vi "ShowDetailResult.vi"(8 "error in (no error)":errorcluster caption="错误输入（无错误）", 11 "DataBase in":refnum<class "DataBase.lvclass">) -> (0 "error out":errorcluster caption="错误输出", 3 "DataBase out":refnum<class "DataBase.lvclass">)   [LabVIEW 2019, in "DataBase.lvlib" / "DataBase.lvclass"]
uses:
  DataBase.lvclass
  DataBase.lvclass/DataBase.ctl
  <vilib>/Utility/miscctls.llb/LVRowAndColumnTypeDef.ctl
  <vilib>/Utility/file.llb/Read Delimited Spreadsheet (string).vi
panel:
  out "File Path Indicator":path
  in  "Multicolumn Listbox":i32(listbox)
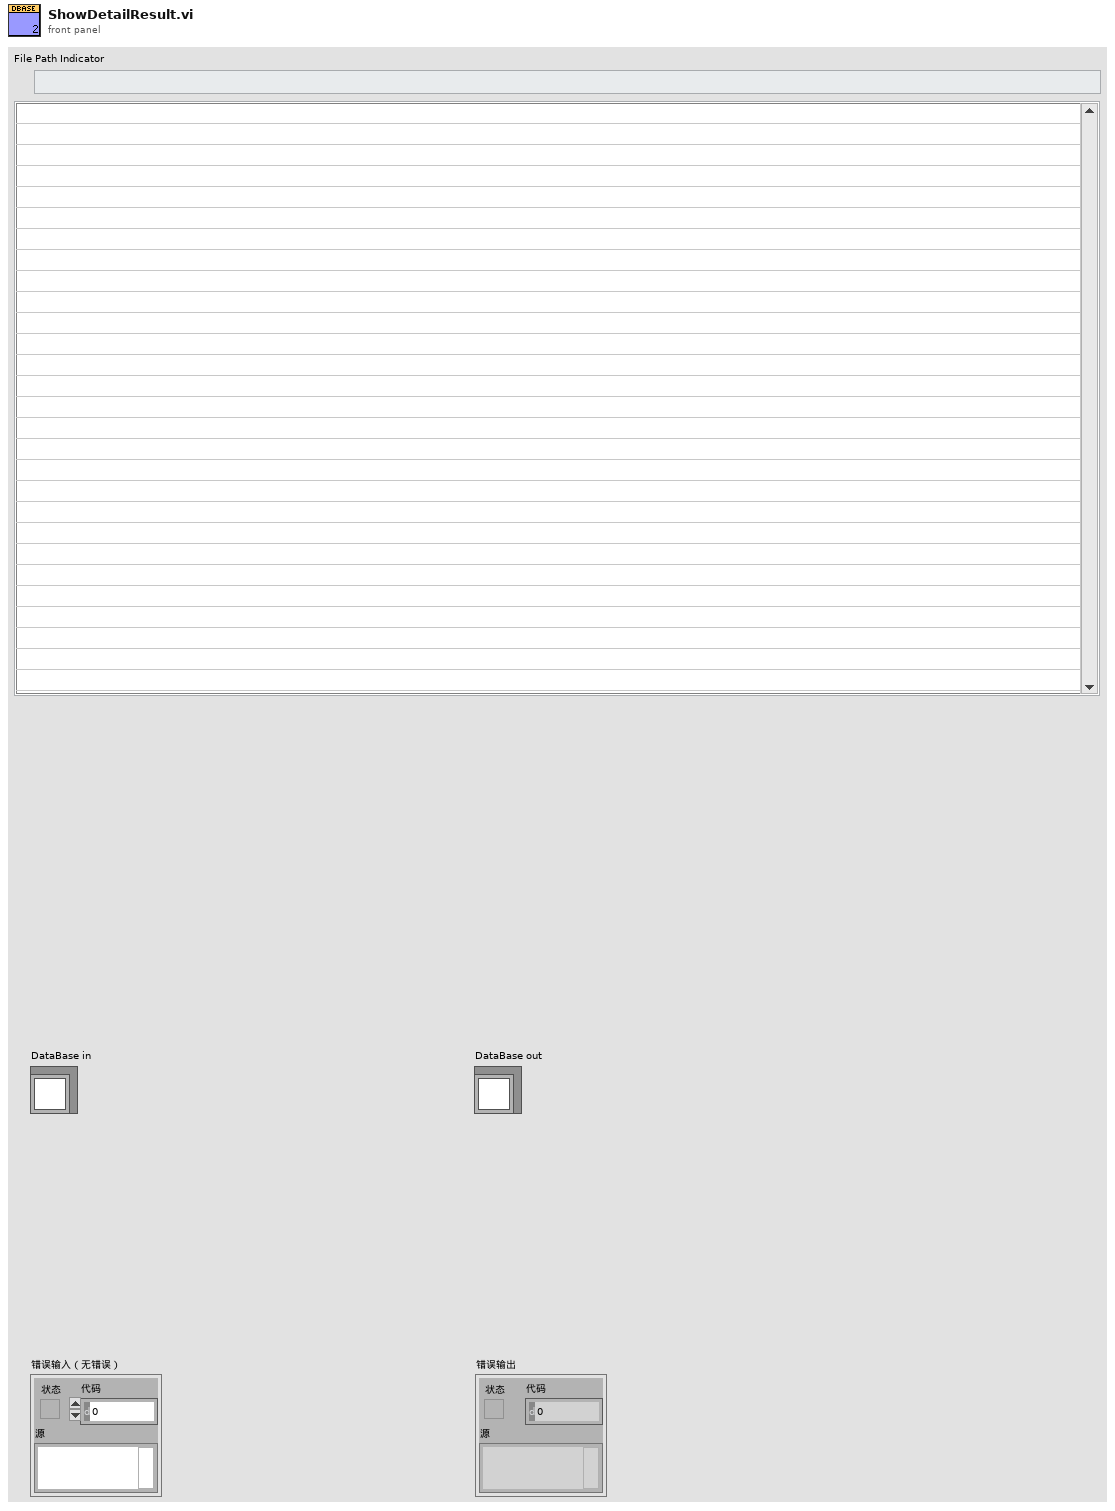
[diagram p1: front panel]
types:
  T1 = enum32{"Invalid", "Standard", "Closed", "Hidden", "Minimized", "Maximized"}
  T2 = enum32{"invalid app kind", "Development System", "Run Time System", "Student Edition", "Embedded LabVIEW", "Evaluation", "Custom"}
  T3 = typedef "LVRowAndColumnTypeDef.ctl" = cluster{"Row":i32, "Column":i32}
  T4 = cluster{"Core":cluster{"Current VI Reference":refnum<vi>, "Close Panel on Exit?":bool}, "Your Boolean data":bool, "Your string data":string, "Multicolumn Listbox":refnum<vi>}
  T5 = cluster{"Current VI Reference":refnum<vi>, "Close Panel on Exit?":bool}
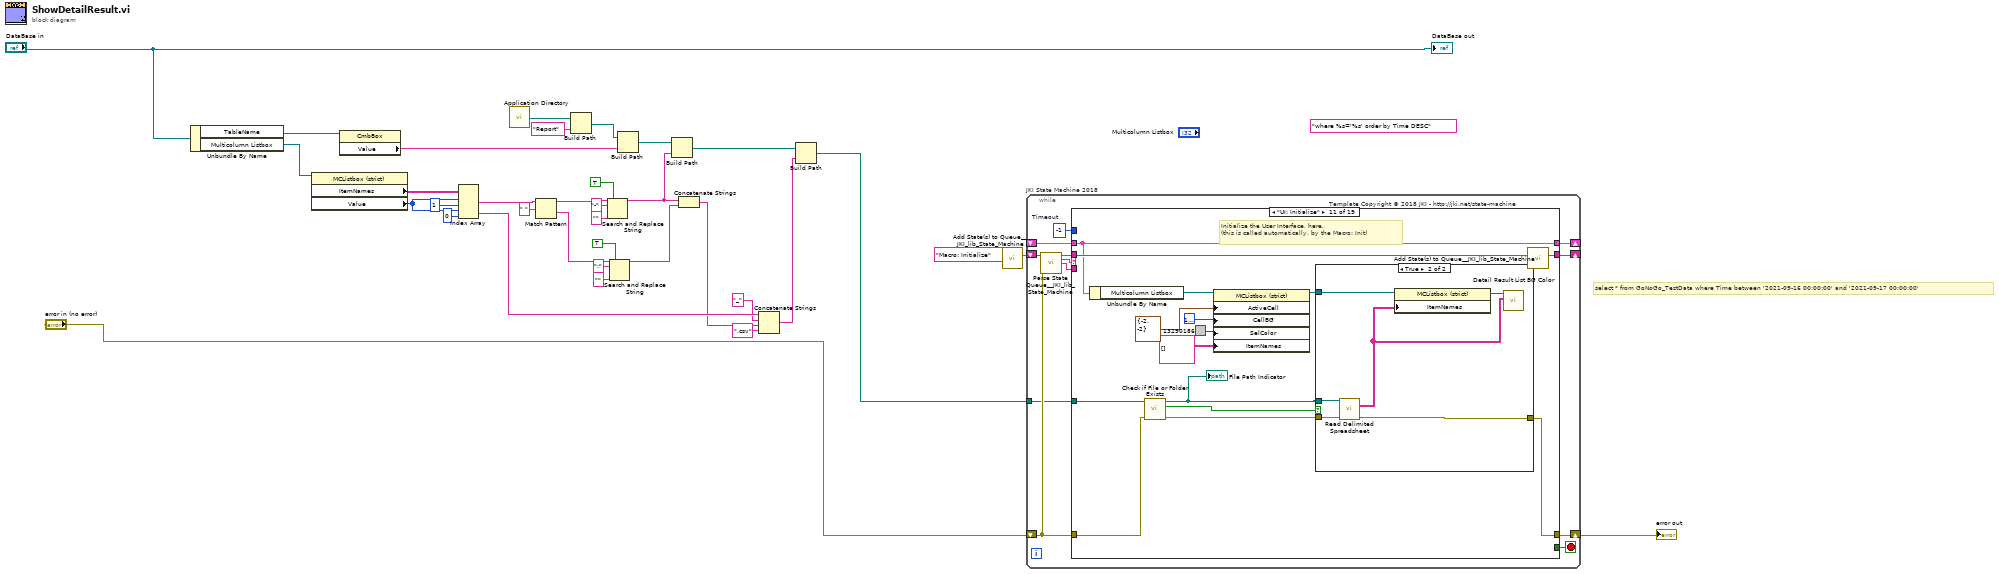
[diagram p0: block diagram]
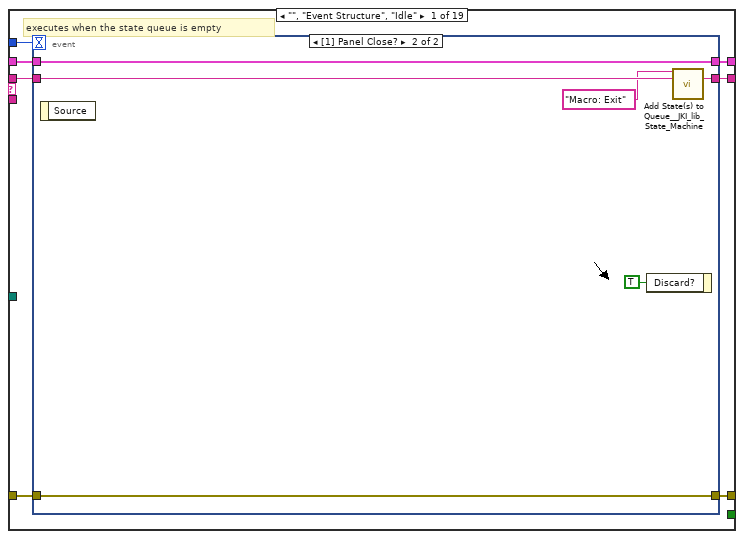
[diagram p2: hidden frame]
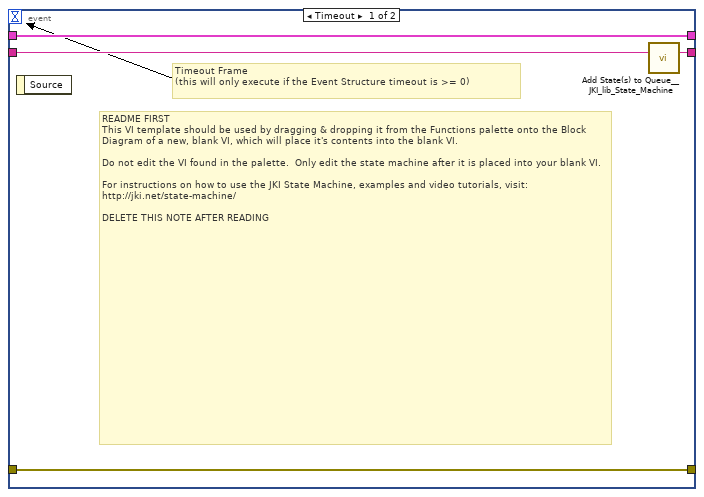
[diagram p3: hidden frame]
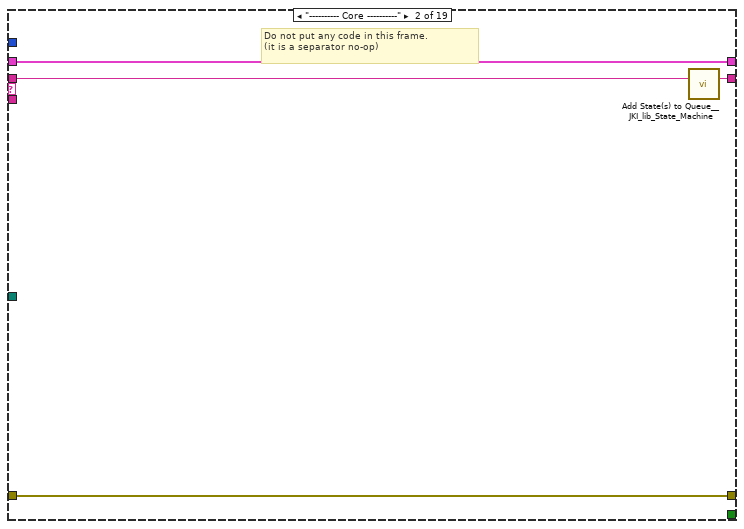
[diagram p4: hidden frame]
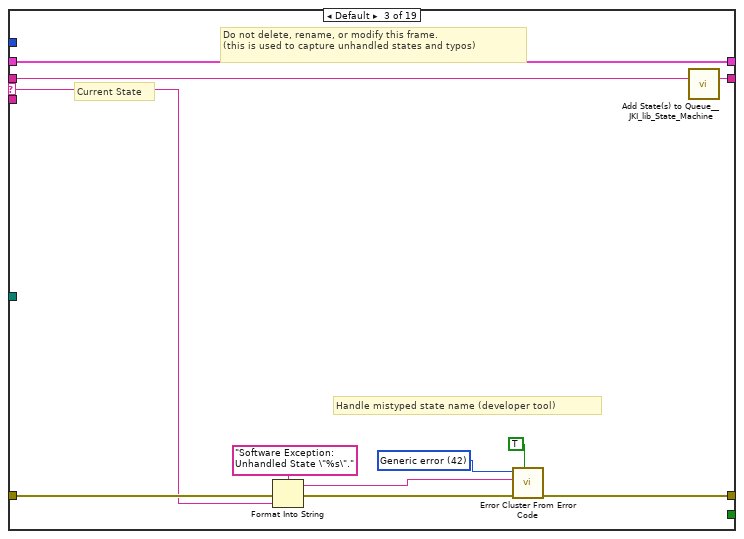
[diagram p5: hidden frame]
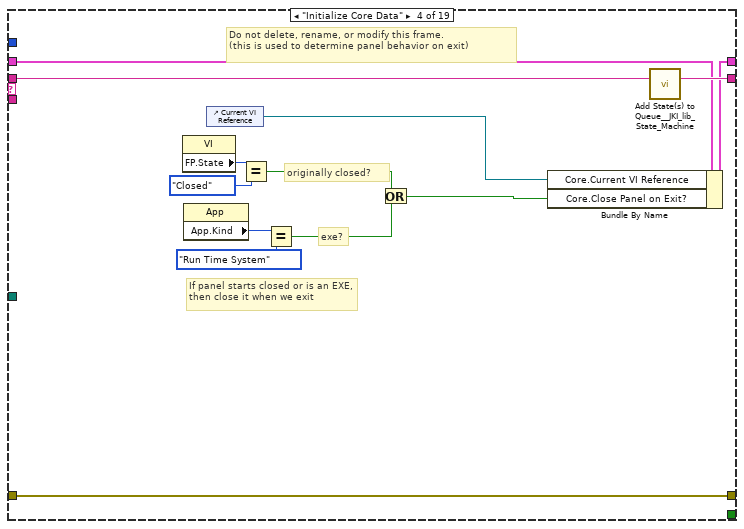
[diagram p6: hidden frame]
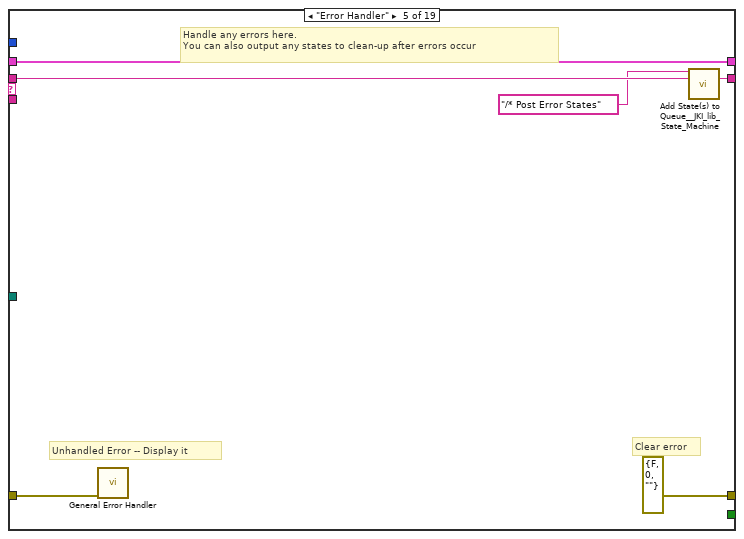
[diagram p7: hidden frame]
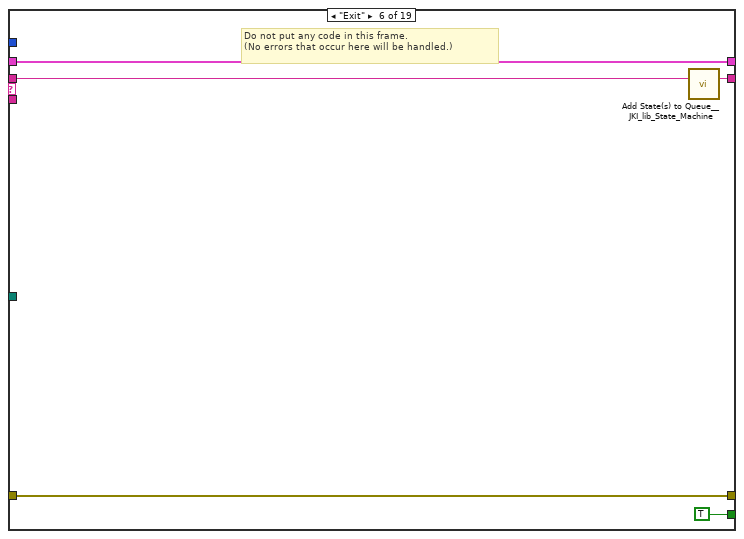
[diagram p8: hidden frame]
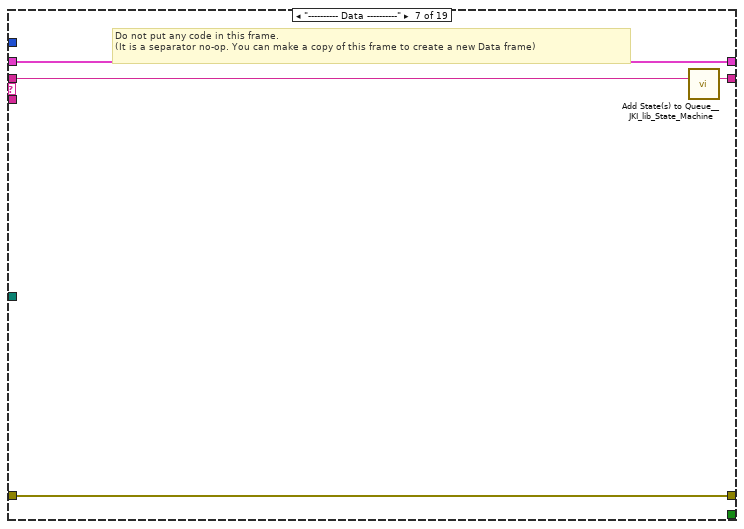
[diagram p9: hidden frame]
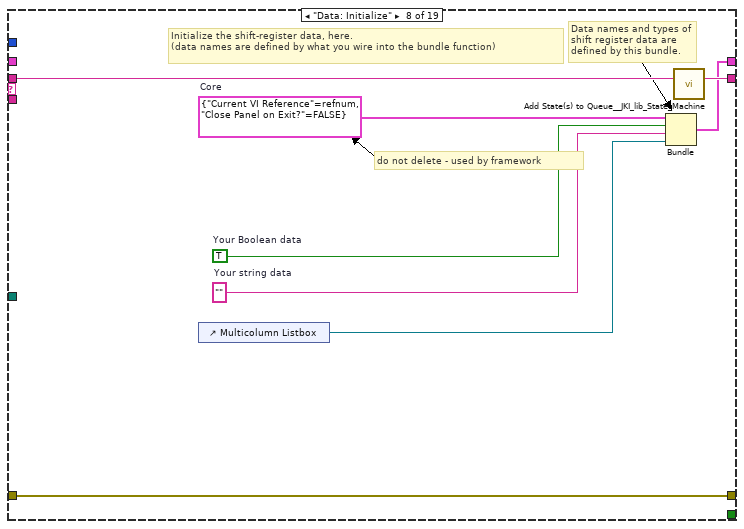
[diagram p10: hidden frame]
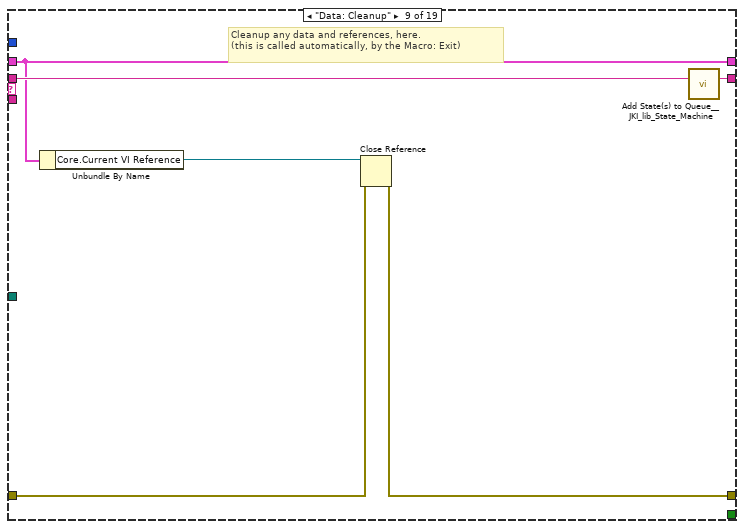
[diagram p11: hidden frame]
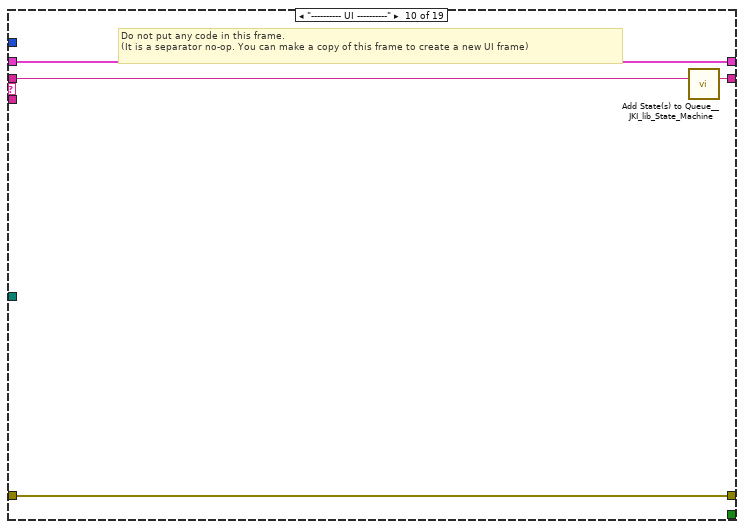
[diagram p12: hidden frame]
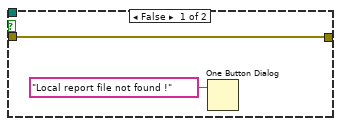
[diagram p13: hidden frame]
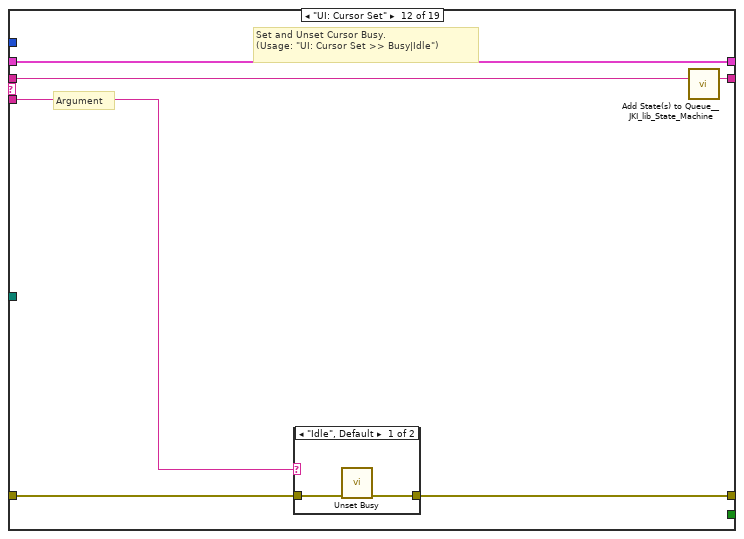
[diagram p14: hidden frame]
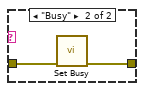
[diagram p15: hidden frame]
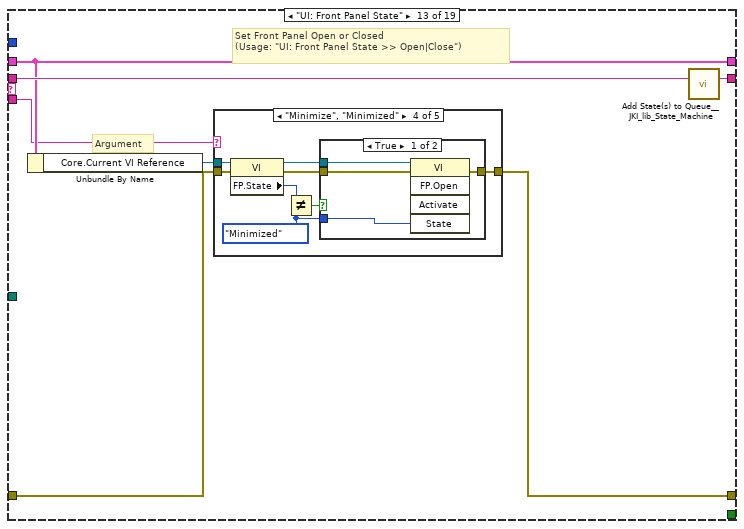
[diagram p16: hidden frame]
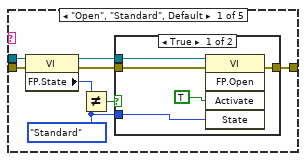
[diagram p17: hidden frame]
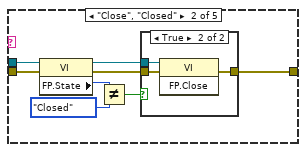
[diagram p19: hidden frame]
diagram:
  (unwired) "where %s='%s' order by Time DESC" ("format string")
  # "select * from GoNoGo_TestData where Time between '2021-09-16 00:00:00' and '2021-09-17 00:00:00'"
  n1 = Unbundle By Name("DataBase in") -> ("TableName"=w32:refnum<vi>, "Multicolumn Listbox"=w26:refnum<vi>)
  n2 = property class="MCListbox (strict)"(reference=w26) -> ("ItemNames"=w25:string[][], "Value"=w16:i32)  [unwired: 1 in, 2 out]
  n3 = property class="CmbBox"(reference=w32) -> ("Value"=w28:string)  [unwired: 1 in, 2 out]
  n4 = Index Array(array=w25, index (row) #1=w16, index (col) #1=1 ("disabled index (col)"), index (row) #2=w16, index (col) #2=0 ("disabled index (col)")) -> (element #1=w22:string, element #2=w8:string)
  n5 = call <vilib>:"Application Directory.vi"() -> ("Application Directory"=w31:path)
  n6 = Match Pattern(string=w22, regular expression=" ") -> (before substring=w21:string, after substring=w11:string)  [unwired: 1 in, 2 out]
  n7 = Build Path(base path=w31, name or relative path="Report") -> (appended path=w30:path)
  n8 = Search and Replace String(replace all?=TRUE ("replace all? (F)"), input string=w21, search string="-", replace string="" ("replace string (\"\")")) -> (result string=w10:string)  [unwired: 4 in, 3 out]
  n9 = Search and Replace String(replace all?=TRUE ("replace all? (F)"), input string=w11, search string=":", replace string="" ("replace string (\"\")")) -> (result string=w9:string)  [unwired: 4 in, 3 out]
  n10 = Build Path(base path=w30, name or relative path=w28) -> (appended path=w27:path)
  n11 = Build Path(base path=w27, name or relative path=w10) -> (appended path=w17:path)
  n12 = Concatenate Strings(w10, w9) -> (w6:string)
  n13 = Concatenate Strings(w8, "_" ("string"), w6, ".csv" ("string")) -> (w4:string)
  n14 = Build Path(base path=w17, name or relative path=w4) -> (appended path=w1:path)
  n15 = call <vilib>:"Add State(s) to Queue__JKI_lib_State_Machine.vi"("State(s) in (\"\")"="Macro: Initialize") -> ("States Out"=w34:string)  [unwired: 14 in]
  n16 = while "JKI State Machine 2018" {
    shift-right: [w40] -> _
    shift-left: _ -> [w39]
    shift-right: [w43] -> w2
    shift-left: "error in (no error)" -> [w37]
    shift-right: [w42] -> _
    shift-left: w34 -> [w44]
    tunnel: w1 -> [w36]
    stop <- w41 stop-if-true
    w38 = -1  # Timeout
    # "Template Copyright © 2018 JKI - http://jki.net/state-machine"
    n17 = call <vilib>:"Parse State Queue__JKI_lib_State_Machine.vi"("State Queue"=w44, "Error In (no error)"=w37) -> ("Remaining States"=w46:string, "Current State"=w47:string, "Arguments"=w45:string)  [unwired: 11 in]
    n18 = case shown="\"UI: Initialize\"" w47 {
      selector: w47 -> [_ _ w69 _ _ _ _ _ _ _ _ _ _ _ _ _ _ _ _]
      tunnel: w46 -> [w54 w68 w73 w92 w98 w103 w107 w115 w121 w125 w140 w154 w165 w234 w239 w249 w253 w257 w261]
      tunnel: w45 -> [_ _ _ _ _ _ _ _ _ _ _ w149 w159 _ _ _ _ _ _]
      tunnel: w39 -> [w52 w65 w71 w85 w95 w101 w104 _ w116 w122 w135 w152 w161 w231 w236 w246 w250 w254 w258]
      tunnel: [w51 w66 w75 w89 errorcluster {"status"=FALSE, "code"=0, "source"=""} ("error out") w100 w105 w112 w117 w123 w132 w150 w162 w232 w237 w247 w251 w255 w259] -> w43
      tunnel: w37 -> [w50 w66 w74 w89 w94 w100 w105 w112 w118 w123 w133 w151 w163 w232 w237 w247 w251 w255 w259]
      tunnel: [w53 w67 w72 w91 w97 w102 w106 w114 w120 w124 w139 w153 w164 w233 w238 w248 w252 w256 w260] -> w42
      tunnel: [_ _ _ _ _ TRUE _ _ _ _ _ _ _ _ _ _ _ _ _] -> w41
      tunnel: [w49 w65 w71 w90 w95 w101 w104 w113 w116 w122 w135 w152 w161 w231 w236 w246 w250 w254 w258] -> w40
      tunnel: w38 -> [w48 _ _ _ _ _ _ _ _ _ _ _ _ _ _ _ _ _ _]
      tunnel: w36 -> [_ _ _ _ _ _ _ _ _ _ w134 _ _ _ _ _ _ _ _]
      frame "", "Event Structure", "Idle" {
        # "executes when the state queue is empty"
        n19 = event shown="[1] Panel Close?" {
          selector: _ -> [_ _]
          dyn-events: _ -> [_ _]
          timeout: w48 -> [_ _]
          tunnel: w54 -> [w58 w64]
          tunnel: [w57 w63] -> w53
          tunnel: w52 -> [w55 w61]
          tunnel: [w56 w62] -> w51
          tunnel: w50 -> [w56 w62]
          tunnel: [w55 w61] -> w49
          event Timeout {
            # "README FIRST\nThis VI template should be used by dragging & dropping it from the Functions palette onto the Block Diagram of a new, blank VI, which will place it's contents into the blank VI.\n\nDo not edit the VI found in the palette.  Only edit the state machine after it is placed into your blank VI.\n\nFor instructions on how to use the JKI State Machine, examples and video tutorials, visit:\nhttp://jki.net/state-machine/\n\nDELETE THIS NOTE AFTER READING"
            # "Timeout Frame\n(this will only execute if the Event Structure timeout is >= 0)"
            n20 = event-data() -> ()  [unwired: 1 in, 1 out]
            n21 = call <vilib>:"Add State(s) to Queue__JKI_lib_State_Machine.vi"("State(s) in (\"\")"=w58) -> ("States Out"=w57:string)  [unwired: 14 in]
          }
          event Panel Close? {
            n22 = event-data() -> ()  [unwired: 1 in, 1 out]
            n23 = event-data("Discard?"=TRUE) -> ()  [unwired: 1 in, 1 out]
            n24 = call <vilib>:"Add State(s) to Queue__JKI_lib_State_Machine.vi"("State(s) in Front (\"\")"="Macro: Exit", "State(s) in (\"\")"=w64) -> ("States Out"=w63:string)  [unwired: 13 in]
          }
        }
      }
      frame "---------- Core ----------" {
        # "Do not put any code in this frame.\n(it is a separator no-op)"
        n25 = call <vilib>:"Add State(s) to Queue__JKI_lib_State_Machine.vi"("State(s) in (\"\")"=w68) -> ("States Out"=w67:string)  [unwired: 14 in]
      }
      frame Default {
        w78 = 42 items=["No error", "Argument error", "Memory is full", "Out of zone", "End of file", "File already open", "Generic file I/O error", "File not found", "File permission error", "Disk is full", "Duplicate path", "Too many files open", "System feature not enabled", "Resource file not found", "Cannot add resource", "Resource not found", "Image not found", "Image memory error", "Pen does not exist", "Config type invalid", "Config token not found", "Config parse error", "Config memory error", "Bad external code format", "Bad external code offset", "External code not present", "Null window", "Destroy window error", "Null menu", "Print aborted", "Bad print record", "Print driver error", "Windows error during printing", "Memory error during printing", "Print dialog error", "Generic print error", "Invalid device refnum", "Device not found", "Device parameter error", "Device unit error", "Cannot open device", "Device call aborted", "Generic error", "Cancelled by user", "Object ID too low", "Object ID too high", "Object not in heap", "Unknown heap", "Unknown object (invalid DefProc)", "Unknown object (DefProc not in table)", "Message out of range", "Invalid (null) method", "Unknown message", "Manager call not supported", "Bad address", "Network operation in progress", "Network operation timed out", "Connection is busy", "Network attribute not supported", "Network error", "Address in use", "System out of memory", "Connection aborted", "Connection refused", "Not connected", "Already connected", "Connection closed", "Initialization error (interapplication manager)", "Bad occurrence", "Wait on unbound occurrence handler", "Occurrence queue overflow", "Datalog type conflict", "Unused", "Unrecognized type (interapplication manager)", "Memory corrupt", "Failed to make temporary DLL", "Old CIN version", "Drag socket not found", "Failed to load drop-object", "Failed to register OLE object", "Failed to release OLE object", "Format specifier type mismatch", "Unknown format specifier", "Too few format specifiers", "Too many format specifiers", "Scan failed", "Newer CIN version", "Error converting to variant", "Runtime menu error", "Password tampered", "Variant attribute not found", "Incompatible variant data type", "Event data is not available", "Event Store is not present", "Occurrence is not found", "Event Queue is not created", "Event info is not available", "Refnum passed is NULL", "Error retrieving Class GUID", "Error retrieving CoClass GUID", "Error retrieving TypeLib GUID.", "Bad built application magic bytes.", "Specific driver is different from the specific driver associated with the Logical Name.", "There is no session opened to the class driver.", "Max Error", "MAX - Error with config objects", "MAX - Error loading configuration", "MAX - Group not supported"]
        # "Current State"
        # "Do not delete, rename, or modify this frame.\n(this is used to capture unhandled states and typos)"
        # "Handle mistyped state name (developer tool)"
        n26 = Format Into String(format string="Software Exception: Unhandled State \"%s\"." ("message"), error in=w74, w69) -> (resulting string=w77:string, error out=w76:errorcluster)  [unwired: 1 in]
        n27 = call <vilib>:"Error Cluster From Error Code.vi"("show call chain? (False)"=TRUE, "error in (no error)"=w76, "error message (\"\")"=w77, "error code (0)"=w78) -> ("error out"=w75:errorcluster)  [unwired: 5 in]
        n28 = call <vilib>:"Add State(s) to Queue__JKI_lib_State_Machine.vi"("State(s) in (\"\")"=w73) -> ("States Out"=w72:string)  [unwired: 14 in]
      }
      frame "Initialize Core Data" {
        # "Do not delete, rename, or modify this frame.\n(this is used to determine panel behavior on exit)"
        # "originally closed?"
        # "exe?"
        # "If panel starts closed or is an EXE, then close it when we exit"
        n29 = property class="VI"() -> ("FP.State"=w82:T1)  [unwired: 2 in, 2 out]
        n30 = property class="App"() -> ("App.Kind"=w88:T2)  [unwired: 2 in, 2 out]
        n31 = control-ref of="Current VI Reference"() -> (w83:refnum<vi>)
        n32 = Equal?(x=w82, y=T1."Closed" ("Front Panel Window:State")) -> (x = y?=w80:bool)
        n33 = Equal?(x=w88, y=T2."Run Time System" ("Application:Kind")) -> (x = y?=w86:bool)
        n34 = Or(x=w80, y=w86) -> (x .or. y?=w84:bool)
        n35 = Bundle By Name(cluster=w85, "Core.Current VI Reference"=w83, "Core.Close Panel on Exit?"=w84) -> (w90:T4)
        n36 = call <vilib>:"Add State(s) to Queue__JKI_lib_State_Machine.vi"("State(s) in (\"\")"=w92) -> ("States Out"=w91:string)  [unwired: 14 in]
      }
      frame "Error Handler" {
        # "Unhandled Error -- Display it"
        # "Handle any errors here.\nYou can also output any states to clean-up after errors occur"
        # "Clear error"
        n37 = call <vilib>:"General Error Handler.vi"("error in (no error)"=w94) -> ()  [unwired: 10 in, 5 out]
        n38 = call <vilib>:"Add State(s) to Queue__JKI_lib_State_Machine.vi"("State(s) in Front (\"\")"="/* Post Error States", "State(s) in (\"\")"=w98) -> ("States Out"=w97:string)  [unwired: 13 in]
      }
      frame "Exit" {
        # "Do not put any code in this frame.\n(No errors that occur here will be handled.)"
        n39 = call <vilib>:"Add State(s) to Queue__JKI_lib_State_Machine.vi"("State(s) in (\"\")"=w103) -> ("States Out"=w102:string)  [unwired: 14 in]
      }
      frame "---------- Data ----------" {
        # "Do not put any code in this frame.\n(It is a separator no-op. You can make a copy of this frame to create a new Data frame)"
        n40 = call <vilib>:"Add State(s) to Queue__JKI_lib_State_Machine.vi"("State(s) in (\"\")"=w107) -> ("States Out"=w106:string)  [unwired: 14 in]
      }
      frame "Data: Initialize" {
        w109 = T5 {"Current VI Reference"=refnum, "Close Panel on Exit?"=FALSE}  # Core
        w111 = TRUE  # Your Boolean data
        w110 = ""  # Your string data
        # "do not delete - used by framework"
        # "Data names and types of shift register data are defined by this bundle."
        # "Initialize the shift-register data, here.\n(data names are defined by what you wire into the bundle function)"
        n41 = control-ref of="Multicolumn Listbox"() -> (w108:refnum<vi>)
        n42 = Bundle("Core"=w109, "Your Boolean data"=w111, "Your string data"=w110, "Multicolumn Listbox"=w108) -> (w113:T4)  [unwired: 1 in]
        n43 = call <vilib>:"Add State(s) to Queue__JKI_lib_State_Machine.vi"("State(s) in (\"\")"=w115) -> ("States Out"=w114:string)  [unwired: 14 in]
      }
      frame "Data: Cleanup" {
        # "Cleanup any data and references, here.\n(this is called automatically, by the Macro: Exit)"
        n44 = Unbundle By Name(w116) -> ("Core.Current VI Reference"=w119:refnum<vi>)
        n45 = Close Reference(reference=w119, error in (no error)=w118) -> (error out=w117:errorcluster)
        n46 = call <vilib>:"Add State(s) to Queue__JKI_lib_State_Machine.vi"("State(s) in (\"\")"=w121) -> ("States Out"=w120:string)  [unwired: 14 in]
      }
      frame "---------- UI ----------" {
        # "Do not put any code in this frame.\n(It is a separator no-op. You can make a copy of this frame to create a new UI frame)"
        n47 = call <vilib>:"Add State(s) to Queue__JKI_lib_State_Machine.vi"("State(s) in (\"\")"=w125) -> ("States Out"=w124:string)  [unwired: 14 in]
      }
      frame "UI: Initialize" {
        # "Initialize the User Interface, here.\n(this is called automatically, by the Macro: Init)"
        n48 = Unbundle By Name(w135) -> ("Multicolumn Listbox"=w127:refnum<vi>)
        n49 = call <vilib>:"Check if File or Folder Exists.vi"("error in (no error)"=w133, "path"=w134) -> ("error out"=w136:errorcluster, "file or folder exists?"=w137:bool, "dup path"=w138:path)  [unwired: 7 in]
        "File Path Indicator" <- w138
        n50 = property class="MCListbox (strict)"(reference=w127, "ActiveCell"=T3 {"Row"=-2, "Column"=-2} ("Active Cell:Active Cell"), "CellBG"=u32 16777225 ("Text.Text Colors:Text Color"), "SelColor"=u32 13290186 ("Selection Color"), "ItemNames"=string[][] [] ("Item Names")) -> (reference out=w126:refnum<vi>)  [unwired: 1 in, 1 out]
        n51 = case shown="True" w137 {
          tunnel: w138 -> [_ w146]
          tunnel: w136 -> [w142 w147]
          tunnel: [w142 w145] -> w132
          tunnel: w126 -> [_ w148]
          frame False {
            n52 = One Button Dialog(message="Local report file not found !") -> ()  [unwired: 1 in, 1 out]
          }
          frame True {
            n53 = call-poly <vilib>:"Read Delimited Spreadsheet.vi"("file path (dialog if empty)"=w146, "error in (no error)"=w147) -> ("all rows"=w143:string[][], "error out"=w145:errorcluster)  [unwired: 8 in, 4 out]
            n54 = property class="MCListbox (strict)"(reference=w148, "ItemNames"=w143) -> (reference out=w144:refnum<vi>)  [unwired: 1 in, 1 out]
            n55 = call "Detail Result List BG Color.vi"("all rows"=w143, "reference"=w144) -> ()  [unwired: 10 in]
          }
        }
        n56 = call <vilib>:"Add State(s) to Queue__JKI_lib_State_Machine.vi"("State(s) in (\"\")"=w140) -> ("States Out"=w139:string)  [unwired: 14 in]
      }
      frame "UI: Cursor Set" {
        # "Argument"
        # "Set and Unset Cursor Busy.\n(Usage: \"UI: Cursor Set >> Busy|Idle\")"
        n57 = case shown="\"Idle\", Default" w149 {
          tunnel: w151 -> [w156 w158]
          tunnel: [w155 w157] -> w150
          frame "Idle", Default {
            n58 = call <vilib>:"Unset Busy.vi"("error in (no error)"=w156) -> ("error out"=w155:errorcluster)  [unwired: 10 in]
          }
          frame "Busy" {
            n59 = call <vilib>:"Set Busy.vi"("error in (no error)"=w158) -> ("error out"=w157:errorcluster)  [unwired: 9 in, 1 out]
          }
        }
        n60 = call <vilib>:"Add State(s) to Queue__JKI_lib_State_Machine.vi"("State(s) in (\"\")"=w154) -> ("States Out"=w153:string)  [unwired: 14 in]
      }
      frame "UI: Front Panel State" {
        # "Argument"
        # "Set Front Panel Open or Closed\n(Usage: \"UI: Front Panel State >> Open|Close\")"
        n61 = Unbundle By Name(w161) -> ("Core.Current VI Reference"=w160:refnum<vi>)
        n62 = case shown="\"Minimize\", \"Minimized\"" w159 {
          tunnel: w163 -> [w171 w186 w197 w210 w223]
          tunnel: [w173 w187 w199 w212 w225] -> w162
          tunnel: w160 -> [w172 w184 w198 w211 w224]
          frame "Open", "Standard", Default {
            w166 = T1."Standard" ("State")
            n63 = property class="VI"(reference=w172, error in=w171) -> (reference out=w169:refnum<vi>, error out=w170:errorcluster, "FP.State"=w168:T1)
            n64 = Not Equal?(x=w168, y=w166) -> (x != y?=w167:bool)
            n65 = case shown="True" w167 {
              tunnel: [w177 w179] -> w173
              tunnel: w170 -> [w176 w179]
              tunnel: w169 -> [w175 _]
              tunnel: w166 -> [w174 _]
              frame True {
                n66 = invoke class="VI" method="FP.Open"(reference=w175, error in=w176, "Activate"=TRUE, "State"=w174) -> (error out=w177:errorcluster)  [unwired: 1 in, 4 out]
              }
              frame False {
              }
            }
          }
          frame "Close", "Closed" {
            n67 = property class="VI"(reference=w184, error in=w186) -> (reference out=w183:refnum<vi>, error out=w185:errorcluster, "FP.State"=w181:T1)
            n68 = Not Equal?(x=w181, y=T1."Closed" ("Front Panel Window:State")) -> (x != y?=w180:bool)
            n69 = case shown="True" w180 {
              tunnel: [w188 w191] -> w187
              tunnel: w185 -> [w188 w190]
              tunnel: w183 -> [_ w189]
              frame False {
              }
              frame True {
                n70 = invoke class="VI" method="FP.Close"(reference=w189, error in=w190) -> (error out=w191:errorcluster)  [unwired: 1 in, 2 out]
              }
            }
          }
          frame "Hidden", "Hide" {
            w192 = T1."Hidden" ("State")
            n71 = property class="VI"(reference=w198, error in=w197) -> (reference out=w195:refnum<vi>, error out=w196:errorcluster, "FP.State"=w194:T1)
            n72 = Not Equal?(x=w194, y=w192) -> (x != y?=w193:bool)
            n73 = case shown="True" w193 {
              tunnel: [w203 w204] -> w199
              tunnel: w196 -> [w202 w204]
              tunnel: w195 -> [w201 _]
              tunnel: w192 -> [w200 _]
              frame True {
                n74 = invoke class="VI" method="FP.Open"(reference=w201, error in=w202, "State"=w200) -> (error out=w203:errorcluster)  [unwired: 2 in, 4 out]
              }
              frame False {
              }
            }
          }
          frame "Minimize", "Minimized" {
            w205 = T1."Minimized" ("State")
            n75 = property class="VI"(reference=w211, error in=w210) -> (reference out=w208:refnum<vi>, error out=w209:errorcluster, "FP.State"=w207:T1)
            n76 = Not Equal?(x=w207, y=w205) -> (x != y?=w206:bool)
            n77 = case shown="True" w206 {
              tunnel: [w216 w217] -> w212
              tunnel: w209 -> [w215 w217]
              tunnel: w208 -> [w214 _]
              tunnel: w205 -> [w213 _]
              frame True {
                n78 = invoke class="VI" method="FP.Open"(reference=w214, error in=w215, "State"=w213) -> (error out=w216:errorcluster)  [unwired: 2 in, 4 out]
              }
              frame False {
              }
            }
          }
          frame "Maximize", "Maximized" {
            w218 = T1."Maximized" ("State")
            n79 = property class="VI"(reference=w224, error in=w223) -> (reference out=w221:refnum<vi>, error out=w222:errorcluster, "FP.State"=w220:T1)
            n80 = Not Equal?(x=w220, y=w218) -> (x != y?=w219:bool)
            n81 = case shown="True" w219 {
              tunnel: [w229 w230] -> w225
              tunnel: w222 -> [w228 w230]
              tunnel: w221 -> [w227 _]
              tunnel: w218 -> [w226 _]
              frame True {
                n82 = invoke class="VI" method="FP.Open"(reference=w227, error in=w228, "State"=w226) -> (error out=w229:errorcluster)  [unwired: 2 in, 4 out]
              }
              frame False {
              }
            }
          }
        }
        n83 = call <vilib>:"Add State(s) to Queue__JKI_lib_State_Machine.vi"("State(s) in (\"\")"=w165) -> ("States Out"=w164:string)  [unwired: 14 in]
      }
      frame "---------- Macro ----------" {
        # "Do not put any code in this frame.\n(It is a separator no-op. You can make a copy of this frame to create a new Macro frame)"
        n84 = call <vilib>:"Add State(s) to Queue__JKI_lib_State_Machine.vi"("State(s) in (\"\")"=w234) -> ("States Out"=w233:string)  [unwired: 14 in]
      }
      frame "Macro: Initialize" {
        w235 = "Data: Initialize\nInitialize Core Data\nUI: Initialize\nUI: Front Panel State >> Open"  # Data: Initialize Initialize Core Data UI: Initialize UI: Front Panel State >> Open
        # "Initialization Macro\n(This is called once, when the VI starts)"
        n85 = call <vilib>:"Add State(s) to Queue__JKI_lib_State_Machine.vi"("State(s) in Front (\"\")"=w235, "State(s) in (\"\")"=w239) -> ("States Out"=w238:string)  [unwired: 13 in]
      }
      frame "Macro: Exit" {
        # "Exit Macro\n(This is called once, when the VI exits)"
        n86 = Unbundle By Name(w246) -> ("Core.Close Panel on Exit?"=w245:bool)
        n87 = Select(t="UI: Front Panel State >> Close", s=w245, f="") -> (s? t:f=w242:string)
        n88 = call <vilib>:"Add State(s) to Queue__JKI_lib_State_Machine.vi"("State(s) in (\"\")"=w242, "State(s) at Back (\"\")"="Data: Cleanup\nExit") -> ("States Out"=w240:string)  [unwired: 13 in]
        n89 = call <vilib>:"Add State(s) to Queue__JKI_lib_State_Machine.vi"("State(s) in Front (\"\")"=w240, "State(s) in (\"\")"=w249) -> ("States Out"=w248:string)  [unwired: 13 in]
      }
      frame "---------- New Category ----------" {
        # "Template Separator\n(You can make a copy of, or modify, this frame)"
        n90 = call <vilib>:"Add State(s) to Queue__JKI_lib_State_Machine.vi"("State(s) in (\"\")"=w253) -> ("States Out"=w252:string)  [unwired: 14 in]
      }
      frame "New Category: 1" {
        # "Your code here.\n(You can make a copy of, or modify, this frame)"
        n91 = call <vilib>:"Add State(s) to Queue__JKI_lib_State_Machine.vi"("State(s) in (\"\")"=w257) -> ("States Out"=w256:string)  [unwired: 14 in]
      }
      frame "New Category: 2" {
        # "Your code here.\n(You can make a copy of, or modify, this frame)"
        n92 = call <vilib>:"Add State(s) to Queue__JKI_lib_State_Machine.vi"("State(s) in (\"\")"=w261) -> ("States Out"=w260:string)  [unwired: 14 in]
      }
    }
  }
  "error out" <- w2
  "DataBase out" <- "DataBase in"
